vi "calculateFaultIndicators.vi"(8 "ErrorIn":errorcluster, 9 "spectrum info":T1[](array[typedef]) {"x-axis units" items=["Time (s)"=0, "Frequency-CB (Hz)"=1, "Frequency-CPB (Hz)"=1248, "Frequency-Arbitrary (Hz)"=2357, "Quefrency (s)"=2, "Revolutions (rev)"=3, "Order"=4, "Speed (RPM)"=11, "Speed (rad/s)"=21, "Index"=65535]; "weighting filter" items=["Linear", "A-weighting", "B-weighting", "C-weighting", "ITU-R 468-4", "Dolby", "CCITT", "C-message", "Wb", "Wc", "Wd", "We", "Wf", "Wh", "Wj", "Wk", "Wm", "AES17 20 kHz lowpass", "AES17 40 kHz lowpass", "AES17 20 kHz highpass", "AES17 40 kHz highpass"]; "dB reference [EU]" format="%.2f"; "engineering units" items=["custom..."=0, "V"=1, "A"=21, "C"=30, "pC"=31, "s"=32, "-"=29, "Pa"=2, "N"=20, "g"=3, "m/s^2"=4, "m/s"=5, "m"=6, "mm/s"=12, "mm"=13, "micron/s"=14, "micron"=15, "in/s^2"=7, "in/s"=8, "in"=9, "mil/s"=10, "mil"=11, "rad/s^2"=16, "rad/s"=17, "rad"=18, "deg/s^2"=26, "deg/s"=27, "deg"=28, "RPM"=22, "cycle/s^2"=23, "Hz"=24, "cycle"=25, "strain"=19]; "spectral info"."window" items=["None "=0, "Hanning"=1, "Hamming"=2, "Blackman-Harris"=3, "Exact Blackman"=4, "Blackman"=5, "Flat Top"=6, "4 Term B-Harris "=7, "7 Term B-Harris"=8, "Low Sidelobe"=9, "Force - Exponential"=10, "Gaussian"=62]}, 10 "order power spectra":T8(array[cluster]) {"order 0" format="%.2p"; "delta order" format="%.2p"; "magnitude" format="%.2f"}, 11 "AccelerationDataFrames":T10) -> (0 "ErrorOut":errorcluster, 2 "Orders and indicators":T7[](array[typedef]), 3 "Fault Indicators":T9)   [LabVIEW 2019]
uses:
  AccelerationDataFrames.ctl
  calculateFaultIndicatorsVIs/FaultIndicators.ctl
  OrderAndIndicators.ctl
  <vilib>/addons/_NISVFA/_Shared subVIs/Controls/svc_Spectrum Info.ctl
  <vilib>/addons/_NISVFA/_Shared subVIs/Controls/svc_X-Axis Units.ctl
  <vilib>/addons/_NISVFA/_Shared subVIs/Controls/svc_Spectrum Type.ctl
  <vilib>/addons/_NISVFA/_Shared subVIs/Controls/svc_Engineering Units Text Ring.ctl
  <vilib>/addons/_NISVFA/_Shared subVIs/Controls/svc_Weighting Filter Text Ring.ctl
  <vilib>/addons/_NISVFA/_Shared subVIs/Controls/svc_Complimentary Spectrum Units.ctl
  <vilib>/Analysis/5stat.llb/RMS (DBL).vi
  <vilib>/addons/_NISVFA/_Spectrum Processing/SVFA Power in Band (N Ch).vi
  <vilib>/addons/_NISVFA/_Spectrum Processing/SVFA Power in Band (1 Ch).vi
  <vilib>/addons/_NISVFA/_Spectrum Processing/SVFA Get Spectrum Subset.vi
  <vilib>/addons/_NISVFA/_Spectrum Processing/SVFA Get Spectrum Subset (1 Ch).vi
  <vilib>/addons/_NISVFA/_Shared subVIs/Common/svc_Spectrum Units.vi
  <vilib>/addons/_NISVFA/_Spectrum Processing/SVFA Unit Conversion.vi
  <vilib>/addons/_NISVFA/_Spectrum Processing/SVFA Unit Conversion (1 Ch).vi
  <vilib>/dlg_ctls.llb/Space Constant.vi
  <vilib>/addons/_NISVFA/_Spectrum Processing/subVIs/svfa_Conversion Utility (spectrum info).vi
  <vilib>/addons/_NISVFA/_Spectrum Processing/subVIs/svfa_Peak to RMS to Peak2Peak.vi
  <vilib>/addons/_NISVFA/_Spectrum Processing/subVIs/svfa_Mag to Mag2.vi
  <vilib>/addons/_NISVFA/_Spectrum Processing/subVIs/svfa_Linear to dB.vi
  <vilib>/addons/_NISVFA/_Spectrum Processing/subVIs/svfa_dBrefA to dBrefB.vi
  <vilib>/addons/_NISVFA/_Spectrum Processing/subVIs/svfa_Spectrum to Spectral Density.vi
  <vilib>/measure/madcrms.llb/Basic Averaged DC-RMS for 1 Chan.vi
  <vilib>/addons/Digital Filter Design/Process.llb/DFD Filtering (Wfm NChan).vi
  <vilib>/measure/madcrms.llb/Basic Averaged DC-RMS for N Chan.vi
  <vilib>/addons/_NISVFA/_Shared subVIs/Common/svc_Format Value (DBL).vi
  <vilib>/addons/_NISVFA/_Shared subVIs/Common/svc_Engineering Units to Unit Label.vi
  <vilib>/addons/_NISVFA/_Shared subVIs/Common/svc_Surround NonAlpha String with Parentheses.vi
  <vilib>/addons/_NISVFA/_Shared subVIs/Common/svc_Get Weighting Enum and Labels.vi
  <vilib>/addons/_NISVFA/_Shared subVIs/Common/svc_Check Frequency Range in Spectrum.vi
  <vilib>/addons/_NISVFA/_Shared subVIs/Common/svc_Caller VI Returned in Error Source.vi
  <vilib>/addons/_NISVFA/_Shared subVIs/Common/svc_Convert Frequency to Frequency String.vi
  <vilib>/addons/_NISVFA/_Shared subVIs/Common/svc_Build Unit Label for Frequency Range.vi
  <vilib>/addons/_NISVFA/_Shared subVIs/Common/svc_Window Parameters.vi
  <vilib>/addons/_NISVFA/_Spectrum Processing/subVIs/svfa_Spectrum Info Window to windowTd Type Def.vi
  <vilib>/gmath/NI_Gmath.lvlib
  <vilib>/measure/NI_MAPro.lvlib
  <vilib>/Analysis/NI_AALPro.lvlib
  <vilib>/addons/Digital Filter Design/NI_DigFilterLicensed.lvlib
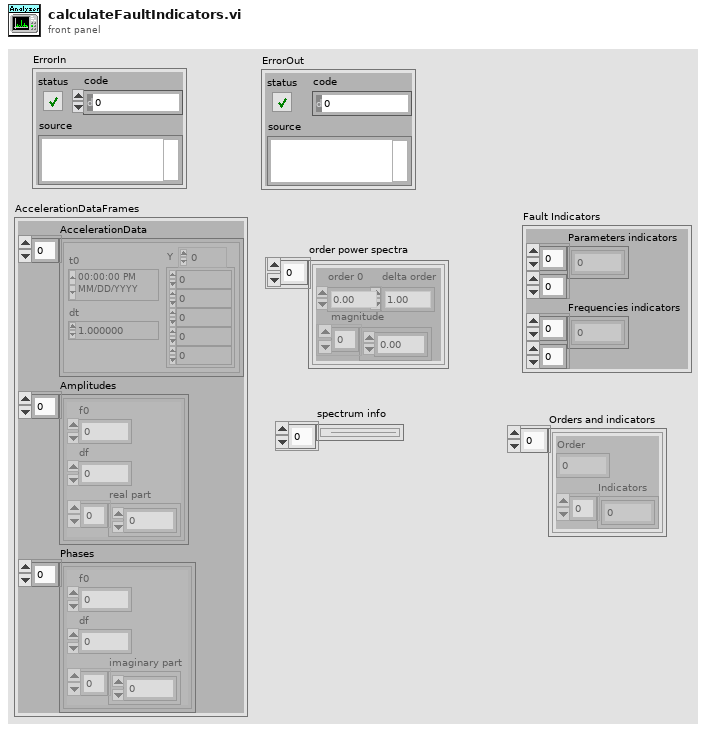
[diagram p1: front panel]
types:
  T1 = typedef "svc_Spectrum Info.ctl" = cluster{"channel name":string, "description":string, "x-axis units":T2, "spectral info":cluster{"spectrum type":T3, "linear/dB":enum16{"linear", "dB"}, "window":u16, "window size":i32, "FFT size":i32}, "engineering units":T4, "custom label":string, "dB reference [EU]":dbl, "peak units":enum16{"rms", "peak", "peak-peak"}, "weighting filter":T5, "spectral density?":bool, "unit label":string, "spectrum skewed?":bool, "complimentary spectrum units":T6}
  T2 = typedef "svc_X-Axis Units.ctl" = u16
  T3 = typedef "svc_Spectrum Type.ctl" = enum16{"FFT Spectrum [complex]", "Amplitude [Magnitude]", "Power [Magnitude^2]", "Cross Spectrum [complex]", "Frequency Response [Complex]"}
  T4 = typedef "svc_Engineering Units Text Ring.ctl" = u16
  T5 = typedef "svc_Weighting Filter Text Ring.ctl" = u16
  T6 = typedef "svc_Complimentary Spectrum Units.ctl" = enum16{"none", "radians", "degrees", "cycles", "imaginary"}
  T7 = typedef "OrderAndIndicators.ctl" = cluster{"Order":dbl, "Indicators":dbl[]}
  T8 = cluster{"order 0":dbl, "delta order":dbl, "magnitude":dbl[]}[]
  T9 = typedef "FaultIndicators.ctl" = cluster{"Parameters indicators":dbl[][], "Frequencies indicators":dbl[][]}
  T10 = typedef "AccelerationDataFrames.ctl" = cluster{"AccelerationData":waveform(dbl)[], "Amplitudes":cluster{"f0":dbl, "df":dbl, "real part":dbl[]}[], "Phases":cluster{"f0":dbl, "df":dbl, "imaginary part":dbl[]}[]}
  T11 = enum16{"Lowpass", "Highpass", "Bandpass", "Bandstop"}
  T12 = typedef "AnalyzerSettings.ctl" = cluster{"Create NS Timeout Code":i32, "Destroy NS Timeout Code":i32, "All threads":T13[], "Connected to app?":bool, "AnalysisSettings":T14}
  T13 = typedef "AThreads.ctl" = enum16{"UI", "analyzeAccelerationData", "aquireAccelerationData", "communicateWebServices", "TDMSmanager", "aquireTachoSignal"}
  T14 = typedef "AnalysisSettings.ctl" = cluster{"Fault Thresholds":T15, "Analysis series name":string, "Save data analysis?":bool, "Band size":i32, "OrderAnalysis?":bool, "Accelerometer":T17, "fs [Hz]":dbl, "Pulse per revolution":u16}
  T15 = typedef "Thresholds.ctl" = cluster{"Parameters labels":T16[], "Parameters thresholds":dbl[], "Freqs and thresholds":dbl[][], "Orders and thresholds":dbl[][]}
  T16 = typedef "FaultParameter.ctl" = enum16{"Kurtosis", "RMS", "Crest factor"}
  T17 = typedef "Accelerometer.ctl" = enum16{"None", "MPU6050", "MMA7351"}
  T18 = typedef "NI_DigFilterLicensed.lvlib/DFD Filter Obj.ctl" = cluster{"mSRate_Fs":dbl, "mSRate_Version":string, "mSRate_Comments":string, "mSRate_OrgCoef":T19, "mSRate_CurCoef":T19, "mSRate_Quantized?":bool, "mSRate_QCoef":T19, "mSRate_QSettings":T21[], "mSRate_Order":i32, "mSRate_Scaling":cluster{"mSRate_ScaleByPowerOf2?":bool, "mSRate_ScaleType":T23}}
  T19 = typedef "NI_DigFilterLicensed.lvlib/DFD Filter Coef.ctl" = cluster{"type":T20, "gain":dbl, "coef a (k)":dbl[], "coef b (v)":dbl[]}
  T20 = typedef "NI_DigFilterLicensed.lvlib/DFD Filter Structure Type Selector.ctl" = enum16{"Undefined", "FIR Direct Form", "FIR Direct Form Transposed", "FIR Symmetric", "FIR Antisymmetric", "IIR Direct Form I", "IIR Direct Form I Transposed", "IIR Direct Form II", "IIR Direct Form II Transposed", "IIR Cascaded Second Order Sections Form I", "IIR Cascaded Second Order Sections Form I Transposed", "IIR Cascaded Second Order Sections Form II", "IIR Cascaded Second Order Sections Form II Transposed", "Lattice Allpass (basic sections)", "Lattice Allpass (one multiplier sections)", "Lattice Allpass (normalized sections)", "Lattice AR (basic sections)", "Lattice AR (one multiplier sections)", "Lattice AR (normalized sections)", "Lattice MA (minimum phase)", "Lattice MA (maximum phase)", "Lattice ARMA (basic sections)", "Lattice ARMA (one multiplier sections)", "Lattice ARMA (normalized sections)"}
  T21 = typedef "NI_DigFilterLicensed.lvlib/dfd_Internal Quantization Settings.ctl" = cluster{"source":T22, "wl":i16, "iwl":i16, "overflow mode":enum16{"Saturation", "Wrap"}, "rounding mode":enum16{"Nearest", "Truncation"}, "signed?":bool}
  T22 = typedef "NI_DigFilterLicensed.lvlib/dfd_Internal Quantization Srcs.ctl" = u16
  T23 = typedef "NI_DigFilterLicensed.lvlib/DFD Coef Norm Type.ctl" = enum16{"No Norm", "Time Domain 1-Norm", "Time Domain 2-Norm", "Time Domain Inf-Norm"}
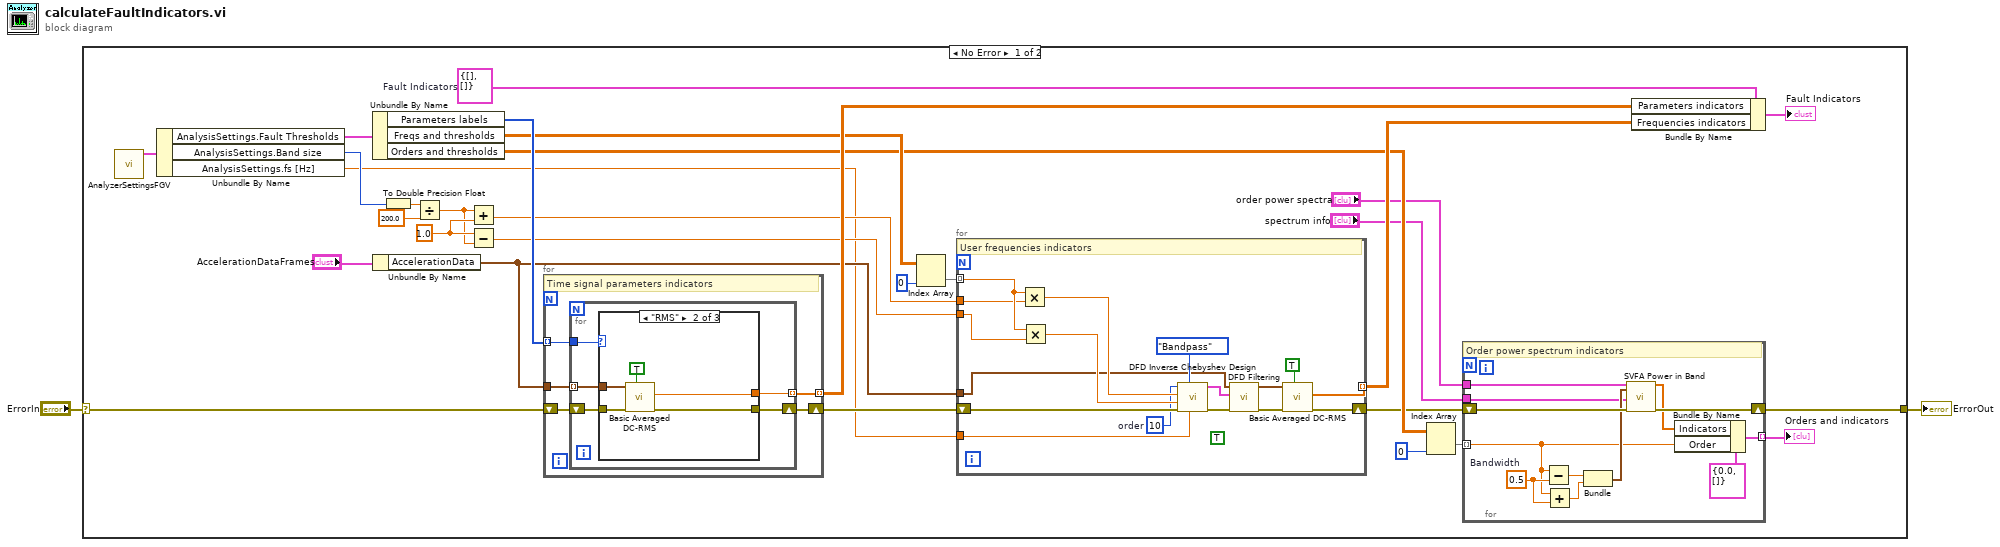
[diagram p0: block diagram]
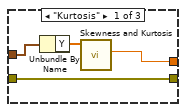
[diagram p2: hidden frame]
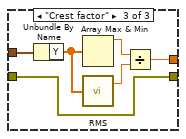
[diagram p3: hidden frame]
diagram:
  n1 = case shown="No Error" "ErrorIn" {
    selector: "ErrorIn" -> [w29 w87]
    tunnel: [w3 w87] -> w1
    frame No Error {
      w12 = 1.0 ("y")
      w32 = T9 {"Parameters indicators"=[], "Frequencies indicators"=[]}  # Fault Indicators
      n2 = call "AnalyzerSettingsFGV.vi"() -> ("AnalyzerSettingsOut"=w17:T12)  [unwired: 11 in]
      n3 = Unbundle By Name(w17) -> ("AnalysisSettings.Fault Thresholds"=w16:T15, "AnalysisSettings.Band size"=w15:i32, "AnalysisSettings.fs [Hz]"=w9:dbl)
      n4 = Unbundle By Name(w16) -> ("Parameters labels"=w30:T16[], "Freqs and thresholds"=w26:dbl[][], "Orders and thresholds"=w8:dbl[][])
      n5 = Unbundle By Name("AccelerationDataFrames") -> ("AccelerationData"=w18:waveform(dbl)[])
      n6 = To Double Precision Float(number=w15) -> (double precision float=w14:dbl)
      n7 = Divide(x=w14, y=200.0) -> (x/y=w11:dbl)
      n8 = Add(x=w11, y=w12) -> (x+y=w22:dbl)
      n9 = Subtract(x=w12, y=w11) -> (x-y=w21:dbl)
      n10 = for {
        tunnel: w18 -> [w66]
        tunnel: w30 -> [w65] mode=indexing
        shift-right: [w63] -> w27
        shift-left: w29 -> [w64]
        tunnel: [w62] -> w28 mode=indexing
        # "Time signal parameters indicators"
        n11 = for {
          tunnel: w66 -> [w71] mode=indexing
          tunnel: [w70] -> w62 mode=indexing
          tunnel: w65 -> [w69]
          shift-right: [w67] -> w63
          shift-left: w64 -> [w68]
          n12 = case shown="\"RMS\"" w69 {
            tunnel: w71 -> [w75 w80 w86]
            tunnel: [w73 w76 w82] -> w70
            tunnel: w68 -> [w72 w78 w81]
            tunnel: [w72 w77 w81] -> w67
            frame "Kurtosis" {
              n13 = Unbundle By Name(w75) -> ("Y"=w74:dbl[])
              n14 = call <vilib>:"Skewness and Kurtosis.vi"("X"=w74) -> ("kurtosis"=w73:dbl)  [unwired: 8 in, 2 out]
            }
            frame "RMS" {
              n15 = call-poly <vilib>:"Basic Averaged DC-RMS.vi"("reset"=TRUE, "error in (no error)"=w78, "signal in"=w80) -> ("error out"=w77:errorcluster, "RMS value"=w76:dbl)  [unwired: 5 in, 2 out]
            }
            frame "Crest factor" {
              n16 = Unbundle By Name(w86) -> ("Y"=w85:dbl[])
              n17 = Array Max & Min(array=w85) -> (max value=w84:dbl)  [unwired: 3 out]
              n18 = call-poly <vilib>:"RMS.vi"("X"=w85) -> ("rms value"=w83:dbl)  [unwired: 1 out]
              n19 = Divide(x=w84, y=w83) -> (x/y=w82:dbl)
            }
          }
        }
      }
      n20 = Index Array(array=w26, index (col)=0 ("disabled index (col)")) -> (element=w24:dbl[])  [unwired: 1 in]
      n21 = for {
        shift-right: [w46] -> w5
        shift-left: w27 -> [w61]
        tunnel: w18 -> [w51]
        tunnel: w24 -> [w60] mode=indexing
        tunnel: [w47] -> w23 mode=indexing
        tunnel: w22 -> [w57]
        tunnel: w21 -> [w56]
        tunnel: w9 -> [w45]
        (unwired) TRUE ("init/cont (init:F)")
        w54 = 10  # order
        # "User frequencies indicators"
        n22 = Multiply(x=w60, y=w57) -> (x*y=w59:dbl)
        n23 = Multiply(x=w60, y=w56) -> (x*y=w58:dbl)
        n24 = call <vilib>:"DFD Inverse Chebyshev Design.vi"("fs [Hz]"=w45, "filter type"=T11."Bandpass", "error in (no error)"=w61, "low cutoff freq [Hz]"=w58, "high cutoff freq [Hz]"=w59, "order"=w54) -> ("error out"=w53:errorcluster, "filter out"=w52:T18)  [unwired: 4 in]
        n25 = call-poly <vilib>:"DFD Filtering.vi"("error in (no error)"=w53, "filter"=w52, "signal in"=w51) -> ("error out"=w49:errorcluster, "signal out"=w50:waveform(dbl)[])  [unwired: 7 in]
        n26 = call-poly <vilib>:"Basic Averaged DC-RMS.vi"("reset"=TRUE, "error in (no error)"=w49, "signals in"=w50) -> ("error out"=w46:errorcluster, "RMS values"=w47:dbl[])  [unwired: 5 in, 2 out]
      }
      n27 = Index Array(array=w8, index (col)=0 ("disabled index (col)")) -> (element=w19:dbl[])  [unwired: 1 in]
      n28 = for {
        shift-right: [w43] -> w3
        shift-left: w5 -> [w44]
        tunnel: w19 -> [w36] mode=indexing
        tunnel: [w37] -> w4 mode=indexing
        tunnel: "order power spectra" -> [w35]
        tunnel: "spectrum info" -> [w34]
        w42 = 0.5  # Bandwidth
        # "Order power spectrum indicators"
        n29 = Subtract(x=w36, y=w42) -> (x-y=w41:dbl)
        n30 = Add(x=w36, y=w42) -> (x+y=w40:dbl)
        n31 = Bundle(w41, w40) -> (w39:cluster{dbl, dbl})  [unwired: 1 in]
        n32 = call-poly <vilib>:"SVFA Power in Band.vi"("spectra"=w35, "range"=w39, "spectrum info"=w34, "error in (no error)"=w44) -> ("powers in band"=w33:dbl[], "error out"=w43:errorcluster)  [unwired: 13 in, 1 out]
        n33 = Bundle By Name(cluster=T7 {"Order"=0.0, "Indicators"=[]} ("Order and indicators"), "Indicators"=w33, "Order"=w36) -> (w37:T7)
      }
      "Orders and indicators" <- w4
      n34 = Bundle By Name(cluster=w32, "Parameters indicators"=w28, "Frequencies indicators"=w23) -> (→"Fault Indicators":T9)
    }
    frame Error {
    }
  }
  "ErrorOut" <- w1
